vi "Main_0.2v.vi"(0 "START":bool) -> ()   [LabVIEW 2016]
uses:
  ctl/config_ctl.ctl
  ctl/force_sensor_data.ctl
  ctl/UI_cmd-ctl.ctl
  ctl/Data_buf_cmd.ctl
  ctl/file_path-cmd.ctl
  Global.vi
panel:
  out "큐의 원소 개수":i32
  out "simulation":bool
  in  "sub_tab":enum32{"graph", "ref", "err"}(tab)=enum."ref"
  in  "Grapb_tap":enum32{"data graph", "sub graph"}(tab)=enum."sub graph"
  out "Strain chart w cal":waveform(dbl)[](graph)
  out "Force chart":waveform(dbl)(graph)
  out "vacuum chart":waveform(dbl)(graph)
  out "Heater chart":i32(graph)=2147483647
  out "Strain raw chart":waveform(dbl)[](graph)=[{"t0"=timestamp(3479370102.41062 s since 1904-01-01), "dt"=0.00062, "Y"=[0.0, 0.0, 0.0, 0.0, 0.0, 0.0, 0.0, 0.0, 0.0, 0.0, 0.0, 0.0, 0.0, 0.0, 0.0, 0.0, 0.0, 0.0, 0.0, 0.0, 0.0, 0.0, 0.0, 0.0, 0.0, 0.0, 0.0, 0.0, 0.0, 0.0, 0.0, 0.0, 0.0, 0.0, 0.0, 0.0, 0.0, 0.0, 0.0, 0.0, 0.0, 0.0, 0.0, 0.0, 0.0, 0.0, 0.0, 0.0, 0.0, 0.0, 0.0, 0.0, 0.0, 0.0, 0.0, 0.0, 0.0, 0.0, 0.0, 0.0, 0.0, 0.0, 0.0, 0.0, 0.0, 0.0, 0.0, 0.0, 0.0, 0.0, 0.0, 0.0, 0.0, 0.0, 0.0, 0.0, 0.0, 0.0, 0.0, 0.0, 0.0, 0.0, 0.0, 0.0, 0.0, 0.0, 0.0, 0.0, 0.0, 0.0, 0.0, 0.0, 0.0, 0.0, 0.0, 0.0, 0.0, 0.0, 0.0, 0.0], "attributes"=variant("NI_ChannelName"=variant(string "변형률_0"), "NI_UnitDescription"=variant(string "Strain"))}, {"t0"=timestamp(3479370102.41062 s since 1904-01-01), "dt"=0.00062, "Y"=[0.0, 0.0, 0.0, 0.0, 0.0, 0.0, 0.0, 0.0, 0.0, 0.0, 0.0, 0.0, 0.0, 0.0, 0.0, 0.0, 0.0, 0.0, 0.0, 0.0, 0.0, 0.0, 0.0, 0.0, 0.0, 0.0, 0.0, 0.0, 0.0, 0.0, 0.0, 0.0, 0.0, 0.0, 0.0, 0.0, 0.0, 0.0, 0.0, 0.0, 0.0, 0.0, 0.0, 0.0, 0.0, 0.0, 0.0, 0.0, 0.0, 0.0, 0.0, 0.0, 0.0, 0.0, 0.0, 0.0, 0.0, 0.0, 0.0, 0.0, 0.0, 0.0, 0.0, 0.0, 0.0, 0.0, 0.0, 0.0, 0.0, 0.0, 0.0, 0.0, 0.0, 0.0, 0.0, 0.0, 0.0, 0.0, 0.0, 0.0, 0.0, 0.0, 0.0, 0.0, 0.0, 0.0, 0.0, 0.0, 0.0, 0.0, 0.0, 0.0, 0.0, 0.0, 0.0, 0.0, 0.0, 0.0, 0.0, 0.0], "attributes"=variant("NI_ChannelName"=variant(string "변형률_1"), "NI_UnitDescription"=variant(string "Strain"))}, {"t0"=timestamp(3479370102.41062 s since 1904-01-01), "dt"=0.00062, "Y"=[0.0, 0.0, 0.0, 0.0, 0.0, 0.0, 0.0, 0.0, 0.0, 0.0, 0.0, 0.0, 0.0, 0.0, 0.0, 0.0, 0.0, 0.0, 0.0, 0.0, 0.0, 0.0, 0.0, 0.0, 0.0, 0.0, 0.0, 0.0, 0.0, 0.0, 0.0, 0.0, 0.0, 0.0, 0.0, 0.0, 0.0, 0.0, 0.0, 0.0, 0.0, 0.0, 0.0, 0.0, 0.0, 0.0, 0.0, 0.0, 0.0, 0.0, 0.0, 0.0, 0.0, 0.0, 0.0, 0.0, 0.0, 0.0, 0.0, 0.0, 0.0, 0.0, 0.0, 0.0, 0.0, 0.0, 0.0, 0.0, 0.0, 0.0, 0.0, 0.0, 0.0, 0.0, 0.0, 0.0, 0.0, 0.0, 0.0, 0.0, 0.0, 0.0, 0.0, 0.0, 0.0, 0.0, 0.0, 0.0, 0.0, 0.0, 0.0, 0.0, 0.0, 0.0, 0.0, 0.0, 0.0, 0.0, 0.0, 0.0], "attributes"=variant("NI_ChannelName"=variant(string "변형률_2"), "NI_UnitDescription"=variant(string "Strain"))}, {"t0"=timestamp(3479370102.41062 s since 1904-01-01), "dt"=0.00062, "Y"=[0.0, 0.0, 0.0, 0.0, 0.0, 0.0, 0.0, 0.0, 0.0, 0.0, 0.0, 0.0, 0.0, 0.0, 0.0, 0.0, 0.0, 0.0, 0.0, 0.0, 0.0, 0.0, 0.0, 0.0, 0.0, 0.0, 0.0, 0.0, 0.0, 0.0, 0.0, 0.0, 0.0, 0.0, 0.0, 0.0, 0.0, 0.0, 0.0, 0.0, 0.0, 0.0, 0.0, 0.0, 0.0, 0.0, 0.0, 0.0, 0.0, 0.0, 0.0, 0.0, 0.0, 0.0, 0.0, 0.0, 0.0, 0.0, 0.0, 0.0, 0.0, 0.0, 0.0, 0.0, 0.0, 0.0, 0.0, 0.0, 0.0, 0.0, 0.0, 0.0, 0.0, 0.0, 0.0, 0.0, 0.0, 0.0, 0.0, 0.0, 0.0, 0.0, 0.0, 0.0, 0.0, 0.0, 0.0, 0.0, 0.0, 0.0, 0.0, 0.0, 0.0, 0.0, 0.0, 0.0, 0.0, 0.0, 0.0, 0.0], "attributes"=variant("NI_ChannelName"=variant(string "변형률_3"), "NI_UnitDescription"=variant(string "Strain"))}]
  out "Strain raw graph":waveform(dbl)[](graph)=[{"t0"=timestamp(3479370102.41062 s since 1904-01-01), "dt"=0.00062, "Y"=[0.04635468247337127, 0.04635468247337127, 0.04635468247337127, 0.04635468247337127, 0.04635468247337127, 0.04635468247337127, 0.04635468247337127, 0.04635468247337127, 0.04635468247337127, 0.04635468247337127, 0.04635468247337127, 0.04635468247337127, 0.04635468247337127, 0.04635468247337127, 0.04635468247337127, 0.04635468247337127, 0.04635468247337127, 0.04635468247337127, 0.04635468247337127, 0.04635468247337127, 0.04635468247337127, 0.04635468247337127, 0.04635468247337127, 0.04635468247337127, 0.04635468247337127, 0.04635468247337127, 0.04635468247337127, 0.04635468247337127, 0.04635468247337127, 0.04635468247337127, 0.04635468247337127, 0.04635468247337127, 0.04635468247337127, 0.04635468247337127, 0.04635468247337127, 0.04635468247337127, 0.04635468247337127, 0.04635468247337127, 0.04635468247337127, 0.04635468247337127, 0.04635468247337127, 0.04635468247337127, 0.04635468247337127, 0.04635468247337127, 0.04635468247337127, 0.04635468247337127, 0.04635468247337127, 0.04635468247337127, 0.04635468247337127, 0.04635468247337127, 0.04635468247337127, 0.04635468247337127, 0.04635468247337127, 0.04635468247337127, 0.04635468247337127, 0.04635468247337127, 0.04635468247337127, 0.04635468247337127, 0.04635468247337127, 0.04635468247337127, 0.04635468247337127, 0.04635468247337127, 0.04635468247337127, 0.04635468247337127, 0.04635468247337127, 0.04635468247337127, 0.04635468247337127, 0.04635468247337127, 0.04635468247337127, 0.04635468247337127, 0.04635468247337127, 0.04635468247337127, 0.04635468247337127, 0.04635468247337127, 0.04635468247337127, 0.04635468247337127, 0.04635468247337127, 0.04635468247337127, 0.04635468247337127, 0.04635468247337127, 0.04635468247337127, 0.04635468247337127, 0.04635468247337127, 0.04635468247337127, 0.04635468247337127, 0.04635468247337127, 0.04635468247337127, 0.04635468247337127, 0.04635468247337127, 0.04635468247337127, 0.04635468247337127, 0.04635468247337127, 0.04635468247337127, 0.04635468247337127, 0.04635468247337127, 0.04635468247337127, 0.04635468247337127, 0.04635468247337127, 0.04635468247337127, 0.04635468247337127], "attributes"=variant("NI_ChannelName"=variant(string "변형률_0"), "NI_UnitDescription"=variant(string "Strain"))}, {"t0"=timestamp(3479370102.41062 s since 1904-01-01), "dt"=0.00062, "Y"=[0.04702815089622699, 0.04702815089622699, 0.04702815089622699, 0.04702815089622699, 0.04702815089622699, 0.04702815089622699, 0.04702815089622699, 0.04702815089622699, 0.04702815089622699, 0.04702815089622699, 0.04702815089622699, 0.04702815089622699, 0.04702815089622699, 0.04702815089622699, 0.04702815089622699, 0.04702815089622699, 0.04702815089622699, 0.04702815089622699, 0.04702815089622699, 0.04702815089622699, 0.04702815089622699, 0.04702815089622699, 0.04702815089622699, 0.04702815089622699, 0.04702815089622699, 0.04702815089622699, 0.04702815089622699, 0.04702815089622699, 0.04702815089622699, 0.04702815089622699, 0.04702815089622699, 0.04702815089622699, 0.04702815089622699, 0.04702815089622699, 0.04702815089622699, 0.04702815089622699, 0.04702815089622699, 0.04702815089622699, 0.04702815089622699, 0.04702815089622699, 0.04702815089622699, 0.04702815089622699, 0.04702815089622699, 0.04702815089622699, 0.04702815089622699, 0.04702815089622699, 0.04702815089622699, 0.04702815089622699, 0.04702815089622699, 0.04702815089622699, 0.04702815089622699, 0.04702815089622699, 0.04702815089622699, 0.04702815089622699, 0.04702815089622699, 0.04702815089622699, 0.04702815089622699, 0.04702815089622699, 0.04702815089622699, 0.04702815089622699, 0.04702815089622699, 0.04702815089622699, 0.04702815089622699, 0.04702815089622699, 0.04702815089622699, 0.04702815089622699, 0.04702815089622699, 0.04702815089622699, 0.04702815089622699, 0.04702815089622699, 0.04702815089622699, 0.04702815089622699, 0.04702815089622699, 0.04702815089622699, 0.04702815089622699, 0.04702815089622699, 0.04702815089622699, 0.04702815089622699, 0.04702815089622699, 0.04702815089622699, 0.04702815089622699, 0.04702815089622699, 0.04702815089622699, 0.04702815089622699, 0.04702815089622699, 0.04702815089622699, 0.04702815089622699, 0.04702815089622699, 0.04702815089622699, 0.04702815089622699, 0.04702815089622699, 0.04702815089622699, 0.04702815089622699, 0.04702815089622699, 0.04702815089622699, 0.04702815089622699, 0.04702815089622699, 0.04702815089622699, 0.04702815089622699, 0.04702815089622699], "attributes"=variant("NI_ChannelName"=variant(string "변형률_1"), "NI_UnitDescription"=variant(string "Strain"))}, {"t0"=timestamp(3479370102.41062 s since 1904-01-01), "dt"=0.00062, "Y"=[0.046751224408544026, 0.046751224408544026, 0.046751224408544026, 0.046751224408544026, 0.046751224408544026, 0.046751224408544026, 0.046751224408544026, 0.046751224408544026, 0.046751224408544026, 0.046751224408544026, 0.046751224408544026, 0.046751224408544026, 0.046751224408544026, 0.046751224408544026, 0.046751224408544026, 0.046751224408544026, 0.046751224408544026, 0.046751224408544026, 0.046751224408544026, 0.046751224408544026, 0.046751224408544026, 0.046751224408544026, 0.046751224408544026, 0.046751224408544026, 0.046751224408544026, 0.046751224408544026, 0.046751224408544026, 0.046751224408544026, 0.046751224408544026, 0.046751224408544026, 0.046751224408544026, 0.046751224408544026, 0.046751224408544026, 0.046751224408544026, 0.046751224408544026, 0.046751224408544026, 0.046751224408544026, 0.046751224408544026, 0.046751224408544026, 0.046751224408544026, 0.046751224408544026, 0.046751224408544026, 0.046751224408544026, 0.046751224408544026, 0.046751224408544026, 0.046751224408544026, 0.046751224408544026, 0.046751224408544026, 0.046751224408544026, 0.046751224408544026, 0.046751224408544026, 0.046751224408544026, 0.046751224408544026, 0.046751224408544026, 0.046751224408544026, 0.046751224408544026, 0.046751224408544026, 0.046751224408544026, 0.046751224408544026, 0.046751224408544026, 0.046751224408544026, 0.046751224408544026, 0.046751224408544026, 0.046751224408544026, 0.046751224408544026, 0.046751224408544026, 0.046751224408544026, 0.046751224408544026, 0.046751224408544026, 0.046751224408544026, 0.046751224408544026, 0.046751224408544026, 0.046751224408544026, 0.046751224408544026, 0.046751224408544026, 0.046751224408544026, 0.046751224408544026, 0.046751224408544026, 0.046751224408544026, 0.046751224408544026, 0.046751224408544026, 0.046751224408544026, 0.046751224408544026, 0.046751224408544026, 0.046751224408544026, 0.046751224408544026, 0.046751224408544026, 0.046751224408544026, 0.046751224408544026, 0.046751224408544026, 0.046751224408544026, 0.046751224408544026, 0.046751224408544026, 0.046751224408544026, 0.046751224408544026, 0.046751224408544026, 0.046751224408544026, 0.046751224408544026, 0.046751224408544026, 0.046751224408544026], "attributes"=variant("NI_ChannelName"=variant(string "변형률_2"), "NI_UnitDescription"=variant(string "Strain"))}, {"t0"=timestamp(3479370102.41062 s since 1904-01-01), "dt"=0.00062, "Y"=[0.04725649492680068, 0.04725649492680068, 0.04725649492680068, 0.04725649492680068, 0.04725649492680068, 0.04725649492680068, 0.04725649492680068, 0.04725649492680068, 0.04725649492680068, 0.04725649492680068, 0.04725649492680068, 0.04725649492680068, 0.04725649492680068, 0.04725649492680068, 0.04725649492680068, 0.04725649492680068, 0.04725649492680068, 0.04725649492680068, 0.04725649492680068, 0.04725649492680068, 0.04725649492680068, 0.04725649492680068, 0.04725649492680068, 0.04725649492680068, 0.04725649492680068, 0.04725649492680068, 0.04725649492680068, 0.04725649492680068, 0.04725649492680068, 0.04725649492680068, 0.04725649492680068, 0.04725649492680068, 0.04725649492680068, 0.04725649492680068, 0.04725649492680068, 0.04725649492680068, 0.04725649492680068, 0.04725649492680068, 0.04725649492680068, 0.04725649492680068, 0.04725649492680068, 0.04725649492680068, 0.04725649492680068, 0.04725649492680068, 0.04725649492680068, 0.04725649492680068, 0.04725649492680068, 0.04725649492680068, 0.04725649492680068, 0.04725649492680068, 0.04725649492680068, 0.04725649492680068, 0.04725649492680068, 0.04725649492680068, 0.04725649492680068, 0.04725649492680068, 0.04725649492680068, 0.04725649492680068, 0.04725649492680068, 0.04725649492680068, 0.04725649492680068, 0.04725649492680068, 0.04725649492680068, 0.04725649492680068, 0.04725649492680068, 0.04725649492680068, 0.04725649492680068, 0.04725649492680068, 0.04725649492680068, 0.04725649492680068, 0.04725649492680068, 0.04725649492680068, 0.04725649492680068, 0.04725649492680068, 0.04725649492680068, 0.04725649492680068, 0.04725649492680068, 0.04725649492680068, 0.04725649492680068, 0.04725649492680068, 0.04725649492680068, 0.04725649492680068, 0.04725649492680068, 0.04725649492680068, 0.04725649492680068, 0.04725649492680068, 0.04725649492680068, 0.04725649492680068, 0.04725649492680068, 0.04725649492680068, 0.04725649492680068, 0.04725649492680068, 0.04725649492680068, 0.04725649492680068, 0.04725649492680068, 0.04725649492680068, 0.04725649492680068, 0.04725649492680068, 0.04725649492680068, 0.04725649492680068], "attributes"=variant("NI_ChannelName"=variant(string "변형률_3"), "NI_UnitDescription"=variant(string "Strain"))}]
  out "Filtered force graph":waveform(dbl)[](graph)
  out "Force graph T":waveform(dbl)(graph)={"t0"=timestamp(0 s since 1904-01-01), "dt"=0.00062, "Y"=array[3100 elements]}
  out "Balance xy T_p":cluster{"X":dbl, "Y":dbl}[](graph)=[{"X"=-5.263322791327499, "Y"=0.7308526066053755}]
  out "ROI intensity":dbl[][](graph)=[[nan, nan, nan, nan], [nan, nan, nan, nan]]
  out "error out UI":errorcluster caption="error out"
  in  "Data load":bool
  in  "Nulling":bool
  in  "pause":bool
  in  "Main_tap":T1(tab)
  in  "Balance_y":dbl(slide) scale=-50.0..50.0
  in  "Balance_x":dbl(slide) scale=-50.0..50.0
  in  "collet on/off":bool=TRUE
  out "Vacuum":dbl(knob)=27.578726717744516 scale=-10.0..80.0
  out "PCB temp":dbl[](array[slide])=[84.21052631578948, 126.31578947368422, 126.31578947368422, 126.31578947368422, 90.0, 84.21052631578948] scale=0.0..200.0
  in  "PCB config":u16(ring)=5
  in  "Zoom":bool
  out "Forece zoom Graph":dbl[](graph)
  out "simulation status":u32(slide) scale=0.0..565.1360644575578
  in  "Simulation config":cluster{"Raw data file path":path, "speed":u32}={"Raw data file path"=path "C:/FDCdata/data/*.dat", "speed"=10} {"speed" scale=0.0..100.0}
  out "Force graph T":waveform(dbl)(graph)={"t0"=timestamp(0 s since 1904-01-01), "dt"=0.00062, "Y"=array[4800 elements]}
  out "trigger":bool
  out "Pickup force":dbl=98.25510170952174 caption="Pickup force (g)" format="%.1f"
  out "Pickup time":dbl=100.0 caption="Pickup time (ms)" format="%.1f"
  in  "Status":string="\r\n15:48:53 - system ini start\r\n15:48:53 - system ini finish\r\n15:48:55 - cam ini\r\n15:49:19 - cam start\r\n15:49:20 - Program stop\r\n15:49:20 - cam stop"
  out "Balance xy rt":cluster{"X":dbl, "Y":dbl}[](graph)
  out "Bonding force":dbl=992.5036050877534 caption="Bonding force (g)" format="%.1f"
  out "Bonding time":dbl=1024.8600000000001 caption="Bonding time (ms)" format="%.1f"
  out "Heater_rt":dbl=nan caption="Heater (c)" format="%.1f"
  out "Vacuum_rt":dbl=nan caption="Vacuum (kpa)" format="%.1f"
  out "Force rt":dbl=-260.0 caption="Force(g)" format="%.1f"
  out "vacuum T":dbl=36.062310289230055 format="%.1f"
  out "Heater temp T":dbl=85.0 caption="Heater temp (dg)" format="%.1f"
  out "Detach force":dbl=35.0820285944681 caption="Detach force (g)" format="%.1f"
  out "Balance xy T":cluster{"X":dbl, "Y":dbl}[](graph)=[{"X"=-5.263322791327499, "Y"=0.7308526066053755}]
  in  "Graph tap":enum32{"All", "IR"}(tab)
  out "Mixed signal":cluster{"force":dbl, "vacuum":dbl, "temp":dbl}(graph)
  out "IR Image":T2(plugin-control)
  in  "Data_tap":enum32{"Table", "Graph"}(tab)
  out "Data Table":string[][](table)=[["989.722772 ", " 1018.660000 ", " 129.870977 ", " 275.900000 ", " 39.437574 ", " 0.007857", "-0.075730 ", " 0.031476 ", " 0.000000 ", ""], ["1035.064263 ", " 1026.720000 ", " 141.740749 ", " 279.000000 ", " 21.594200 ", " 0.064365", "-0.070932 ", " -0.026859 ", " 0.000000 ", ""], ["953.326654 ", " 1018.040000 ", " 144.008701 ", " 276.520000 ", " 19.439881 ", " 0.048826", "-0.083029 ", " 0.031694 ", " 0.000000 ", ""], ["979.122812 ", " 1027.960000 ", " 140.533487 ", " 275.900000 ", " 17.521738 ", " 0.005569", "-0.069651 ", " 0.008560 ", " 0.000000 ", ""], ["1043.949852 ", " 1042.840000 ", " 134.488977 ", " 275.900000 ", " 13.192071 ", " 0.021168", "-0.072055 ", " 0.031519 ", " 0.000000 ", ""], ["1071.984719 ", " 1048.420000 ", " 138.327061 ", " 275.280000 ", " 25.559397 ", " 0.035083", "-0.035856 ", " -0.018712 ", " 0.000000 ", ""], ["1046.754193 ", " 1028.580000 ", " 142.008722 ", " 275.900000 ", " 18.790541 ", " 0.050977", "-0.061814 ", " 0.072167 ", " 0.000000 ", ""], ["978.664436 ", " 1027.960000 ", " 136.487201 ", " 276.520000 ", " 9.468253 ", " -0.003054", "-0.055865 ", " 0.026074 ", " 0.000000 ", ""], ["976.067518 ", " 1033.540000 ", " 146.571229 ", " 276.520000 ", " 22.608603 ", " 0.020801", "-0.074720 ", " -0.001809 ", " 0.000000 ", ""], ["1056.774276 ", " 1018.660000 ", " 147.195488 ", " 273.420000 ", " 10.587437 ", " 0.032608", "-0.051327 ", " 0.007079 ", " 0.000000 ", ""], ["990.239962 ", " 1018.660000 ", " 112.936811 ", " 270.320000 ", " 42.850519 ", " 0.033952", "-0.070209 ", " 0.070206 ", " 0.000000 ", ""], ["936.169153 ", " 1018.660000 ", " 140.782457 ", " 272.800000 ", " 12.421586 ", " -0.020109", "-0.070449 ", " 0.014964 ", " 0.000000 ", ""], ["941.421956 ", " 1014.320000 ", " 149.172818 ", " 274.660000 ", " 26.213624 ", " -0.007032", "-0.073163 ", " 0.004508 ", " 0.000000 ", ""], ["1034.387749 ", " 1023.000000 ", " 138.956480 ", " 270.940000 ", " 11.759580 ", " 0.086476", "-0.084766 ", " 0.052867 ", " 0.000000 ", ""], ["996.857727 ", " 1021.760000 ", " 157.070597 ", " 274.040000 ", " 25.263497 ", " 0.047311", "-0.063551 ", " 0.014572 ", " 0.000000 ", ""], ["989.722772 ", " 1018.660000 ", " 129.870977 ", " 275.900000 ", " 39.437574 ", " 0.007857", "-0.075730 ", " 0.031476 ", " 0.000000 ", ""], ["1035.064263 ", " 1026.720000 ", " 141.740749 ", " 279.000000 ", " 21.594200 ", " 0.064365", "-0.070932 ", " -0.026859 ", " 0.000000 ", ""], ["953.326654 ", " 1018.040000 ", " 144.008701 ", " 276.520000 ", " 19.439881 ", " 0.048826", "-0.083029 ", " 0.031694 ", " 0.000000 ", ""], ["979.122812 ", " 1027.960000 ", " 140.533487 ", " 275.900000 ", " 17.521738 ", " 0.005569", "-0.069651 ", " 0.008560 ", " 0.000000 ", ""], ["1043.949852 ", " 1042.840000 ", " 134.488977 ", " 275.900000 ", " 13.192071 ", " 0.021168", "-0.072055 ", " 0.031519 ", " 0.000000 ", ""], ["1071.984719 ", " 1048.420000 ", " 138.327061 ", " 275.280000 ", " 25.559397 ", " 0.035083", "-0.035856 ", " -0.018712 ", " 0.000000 ", ""], ["1046.754193 ", " 1028.580000 ", " 142.008722 ", " 275.900000 ", " 18.790541 ", " 0.050977", "-0.061814 ", " 0.072167 ", " 0.000000 ", ""], ["978.664436 ", " 1027.960000 ", " 136.487201 ", " 276.520000 ", " 9.468253 ", " -0.003054", "-0.055865 ", " 0.026074 ", " 0.000000 ", ""], ["976.067518 ", " 1033.540000 ", " 146.571229 ", " 276.520000 ", " 22.608603 ", " 0.020801", "-0.074720 ", " -0.001809 ", " 0.000000 ", ""], ["1056.774276 ", " 1018.660000 ", " 147.195488 ", " 273.420000 ", " 10.587437 ", " 0.032608", "-0.051327 ", " 0.007079 ", " 0.000000 ", ""], ["990.239962 ", " 1018.660000 ", " 112.936811 ", " 270.320000 ", " 42.850519 ", " 0.033952", "-0.070209 ", " 0.070206 ", " 0.000000 ", ""], ["936.169153 ", " 1018.660000 ", " 140.782457 ", " 272.800000 ", " 12.421586 ", " -0.020109", "-0.070449 ", " 0.014964 ", " 0.000000 ", ""], ["941.421956 ", " 1014.320000 ", " 149.172818 ", " 274.660000 ", " 26.213624 ", " -0.007032", "-0.073163 ", " 0.004508 ", " 0.000000 ", ""], ["1034.387749 ", " 1023.000000 ", " 138.956480 ", " 270.940000 ", " 11.759580 ", " 0.086476", "-0.084766 ", " 0.052867 ", " 0.000000 ", ""], ["996.857727 ", " 1021.760000 ", " 157.070597 ", " 274.040000 ", " 25.263497 ", " 0.047311", "-0.063551 ", " 0.014572 ", " 0.000000 ", ""]]
  out "Analysis graph":dbl[](graph)
  out "Data result":cluster{"Mean":dbl, "Max":dbl, "Min":dbl}
  in  "Data menu":T3
  out "balance trend":cluster{"X":dbl, "Y":dbl}[](graph)
  in  "file path":path=path "C:/FDCdata/data/Txt-data_1429_via_simulation.txt" caption="Data file path"
  in  "config tap":enum32{"Program", "etc"}(tab)
  in  "save drive":T4(ring)
  in  "cDAQ config":T5={"sampling rate"=4000.0, "sample to read"=400.0}
  in  "Config":T6={"Lower Cut-Off"=200.0, "Vacuum Trigger level"=20.0, "state settings"={"method"=enum."histogram", "histogram size"=512, "histogram method"=enum."mode", "reserved"=1.0}, "SPA-300 Setting"={"Bonding force (g)"=1000.0, "Bonding time (ms)"=1000.0, "Pickup force (g)"=80.0, "Pickup time (ms)"=200.0, "Speed"=enum."Slow"}, "sensor file"=path ""} {"state settings"."reserved" format="%0.2f"}
  in  "Save_setting":bool
  in  "Load_setting":bool
  out "Force Sensor data":T7={"weight"={"front"=0.28, "left"=0.19, "back"=0.17, "right"=0.36}, "strain map"=[{"x"=-0.0001, "y"=-260.0}, {"x"=0.0, "y"=0.0}, {"x"=0.0001, "y"=260.0}, {"x"=0.000265, "y"=512.0}, {"x"=0.000555, "y"=1042.0}, {"x"=0.00075, "y"=1392.0}, {"x"=0.00082, "y"=1500.0}]}
  out "ROI":T8={"Global Rectangle"=[197, 225, 220, 242], "Contours"=[{"Contour Type"=0, "ROI Type"=3, "Points"=[197, 225, 220, 242]}]}
  in  "정지":bool=TRUE
  # "Real Monitoring"
  # "Balance"
  # "Force"
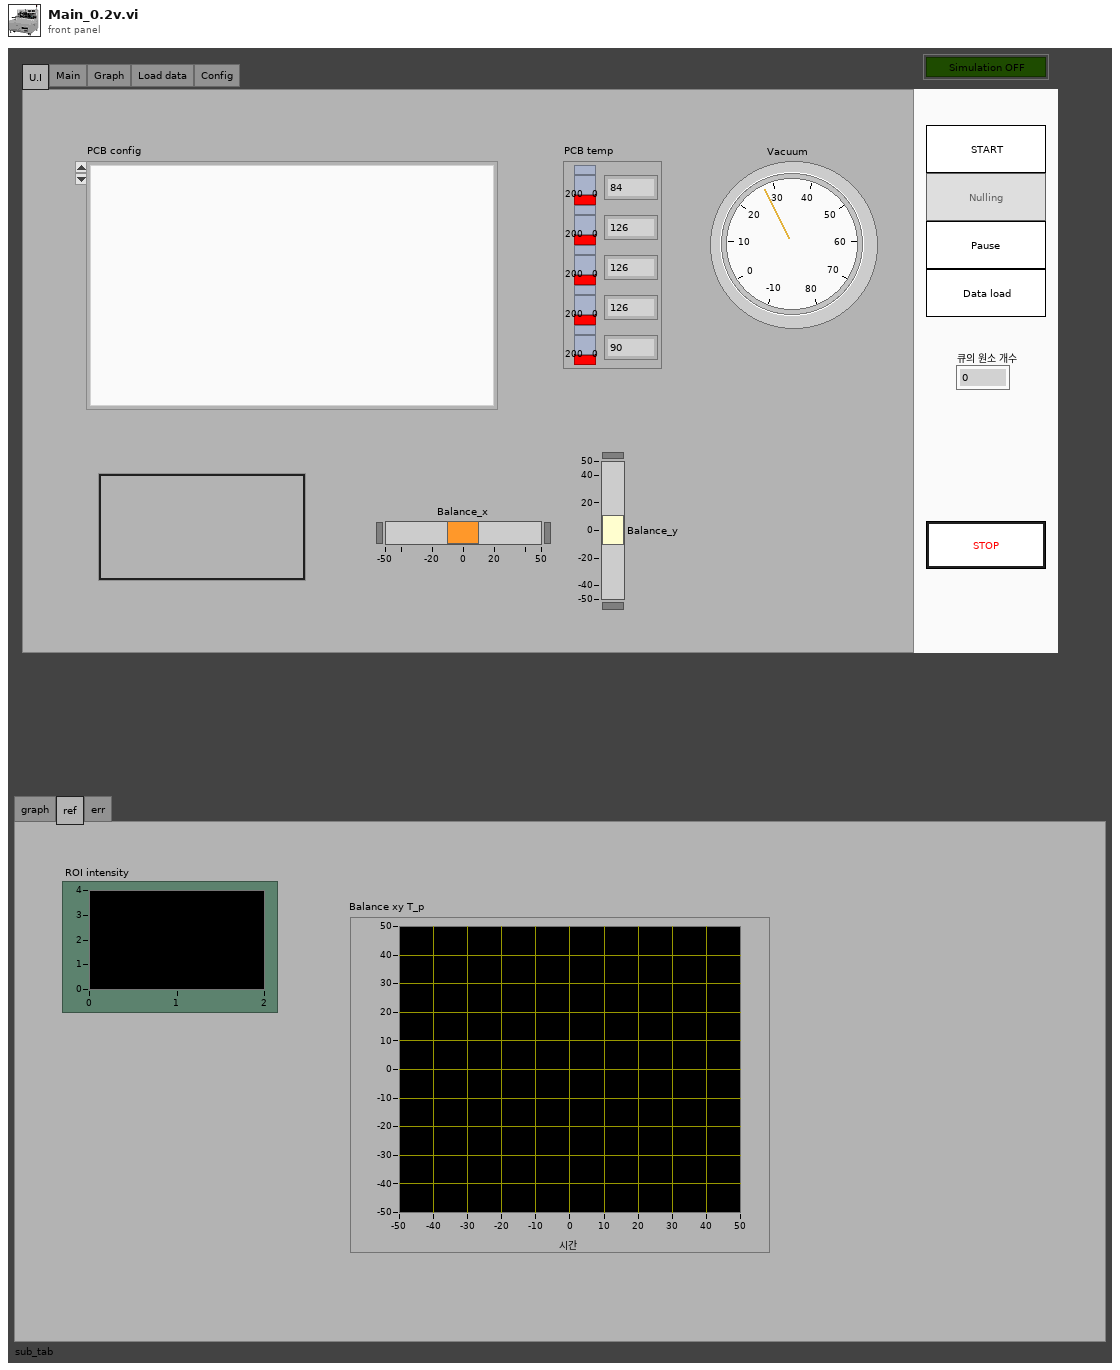
[diagram p1: front panel]
types:
  T1 = enum32{"U.I", "Main", "Graph", "Load data", "Config"}
  T2 = typedef "IMAQ Image.ctl" = refnum<image>
  T3 = cluster{"Force load":bool, "Force load 2":bool, "Force load 3":bool, "Force load 4":bool, "Force load 5":bool, "Force load 8":bool, "Force load 9":bool, "Force load 6":bool, "Force load 7":bool}
  T4 = enum16{"C:\\", "D:\\", "E:\\", "F:\\", "G:\\", "H:\\", "I:\\"}
  T5 = cluster{"sampling rate":dbl, "sample to read":dbl}
  T6 = typedef "config_ctl.ctl" = cluster{"Lower Cut-Off":dbl, "Vacuum Trigger level":dbl, "state settings":cluster{"method":enum32{"histogram", "peak", "auto select"}, "histogram size":i32, "histogram method":enum16{"mode"}, "reserved":dbl}, "SPA-300 Setting":cluster{"Bonding force (g)":dbl, "Bonding time (ms)":dbl, "Pickup force (g)":dbl, "Pickup time (ms)":dbl, "Speed":enum16{"Slow", "Fast"}}, "sensor file":path}
  T7 = typedef "force_sensor_data.ctl" = cluster{"weight":cluster{"front":dbl, "left":dbl, "back":dbl, "right":dbl}, "strain map":cluster{"x":dbl, "y":dbl}[]}
  T8 = cluster{"Global Rectangle":i32[], "Contours":cluster{"Contour Type":u32, "ROI Type":u32, "Points":i32[]}[]}
  T9 = typedef "UI_cmd-ctl.ctl" = enum16{"default", "create", "read"}
  T10 = typedef "Data_buf_cmd.ctl" = enum16{"insert", "default", "create", "clear"}
  T11 = enum8{"Enabled", "Disabled", "Disabled and Grayed Out"}
  T12 = cluster{"PCB temp":refnum<vi>, "Vacuum":refnum<vi>, "PCB config":refnum<vi>, "Balance_x":refnum<vi>, "Balance_y":refnum<vi>}
  T13 = cluster{"Heater temp T":refnum<vi>, "Heater chart":refnum<vi>, "vacuum T":refnum<vi>, "Balance xy rt":refnum<vi>, "Strain chart w cal":refnum<vi>, "Pickup force":refnum<vi>, "Pickup time":refnum<vi>, "Force chart":refnum<vi>, "Force graph T":refnum<vi>, "vacuum chart":refnum<vi>, "vacuum rt":refnum<vi>, "Strain raw graph":refnum<vi>, "Strain raw chart":refnum<vi>, "Bonding time":refnum<vi>, "Bonding force":refnum<vi>, "Balance xy T":refnum<vi>, "Filtered force graph":refnum<vi>, "ROI intensity":refnum<vi>, "Heater_rt":refnum<vi>, "Detach force":refnum<vi>, "Force rt":refnum<vi>, "Mixed signal":refnum<vi>}
  T14 = typedef "q_data.ctl" = cluster{"Strain raw wf":waveform(dbl)[], "vacuum raw wf":waveform(dbl), "IR raw 2d":i16[][]}
  T15 = typedef "log_data.ctl" = cluster{"strain filter_n_nulling wf":waveform(dbl)[], "force wf":waveform(dbl), "force":dbl, "Balance xy wfs":cluster{"X":dbl, "Y":dbl}[], "vacuum kpa wf":waveform(dbl), "pcb temp":dbl[][]}
  T16 = typedef "data.ctl" = cluster{"Bonding force":dbl, "Bonding time":dbl, "Bonding index":dbl, "Pickup force":dbl, "Pickup time":dbl, "Pickup index":dbl, "Detach force":dbl, "Detach time":dbl, "Detach index":dbl, "Heater temp rt":dbl, "Vacuum rt":dbl, "IR raw data":i16[][], "IR temp data":dbl[][], "vacuum raw wf":waveform(dbl), "vacuum kpa wf":waveform(dbl), "strain raw wf":waveform(dbl)[], "Force rt":dbl, "Vacuum T":dbl, "Heater temp T":dbl, "Balance xy arrays":cluster{dbl, dbl}[], "Balance xy":cluster{dbl, dbl}[], "Bonding wf index":dbl, "Pickup wf index":dbl, "Bonding rising index":dbl, "Bonding falling index":dbl, "Pickup rising index":dbl, "Pickup falling index":dbl}
  T17 = typedef "file_path-cmd.ctl" = enum16{"default", "write"}
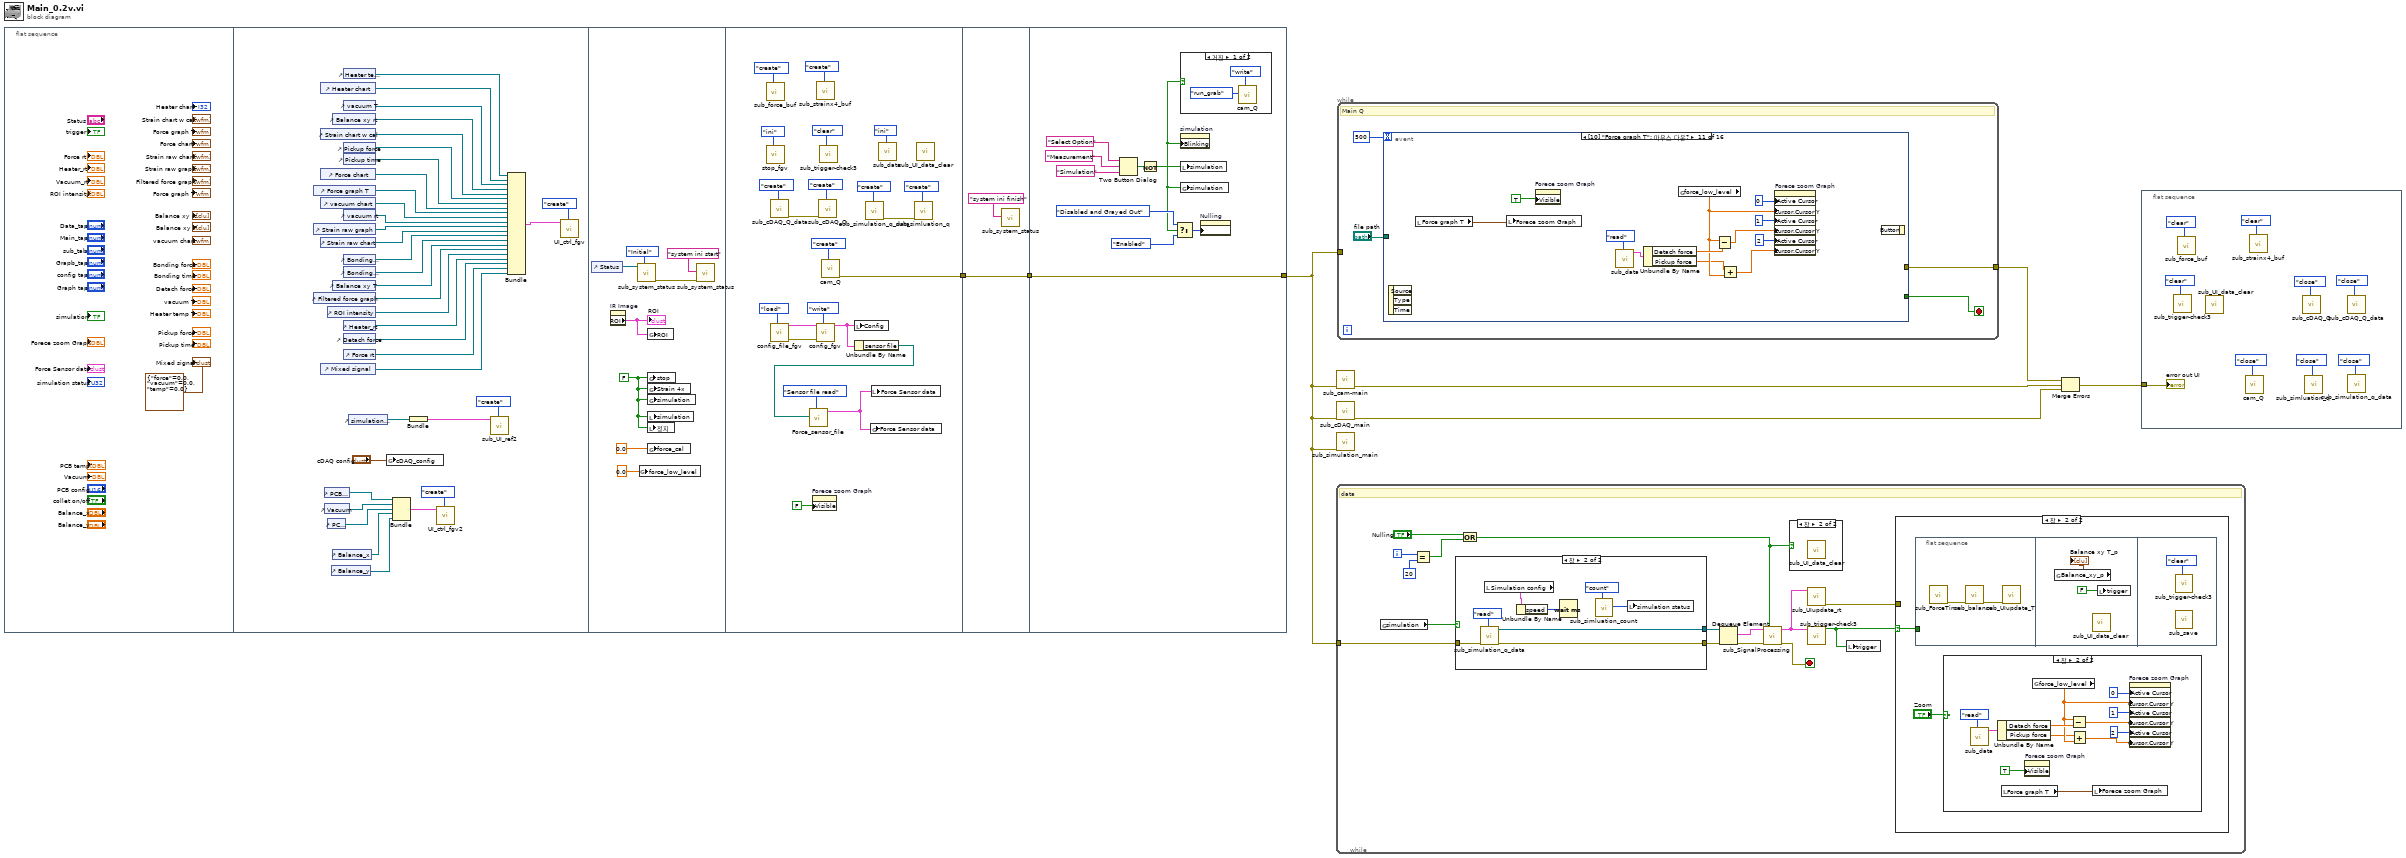
[diagram p0: block diagram]
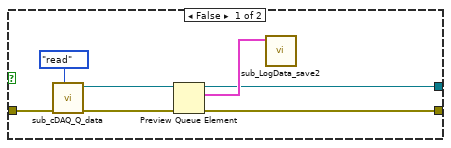
[diagram p2: hidden frame]
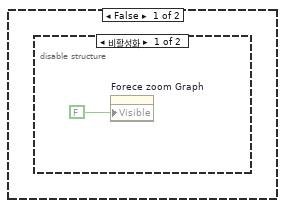
[diagram p5: hidden frame]
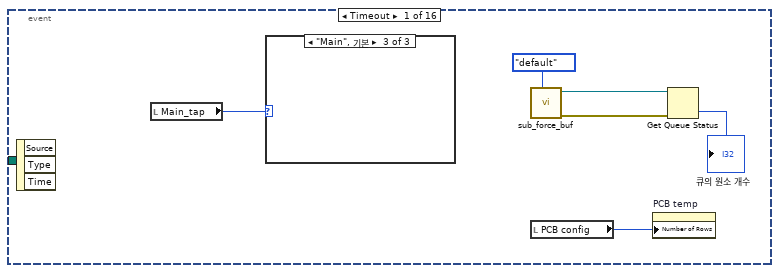
[diagram p7: hidden frame]
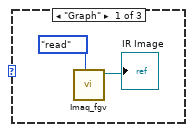
[diagram p8: hidden frame]
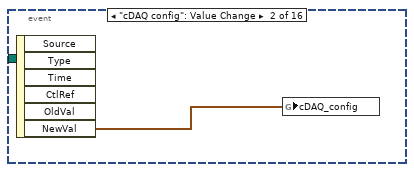
[diagram p10: hidden frame]
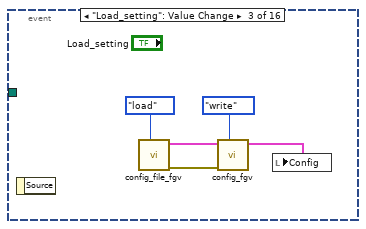
[diagram p11: hidden frame]
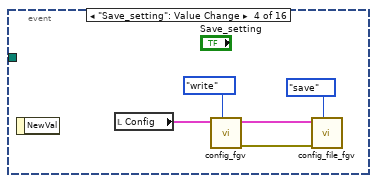
[diagram p12: hidden frame]
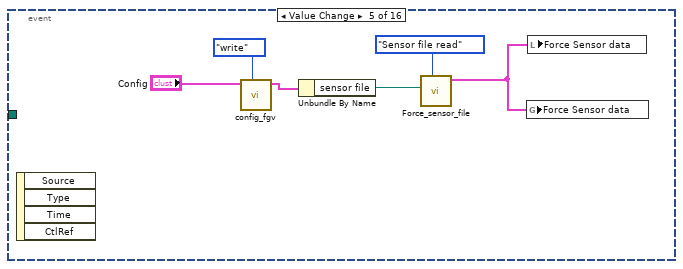
[diagram p13: hidden frame]
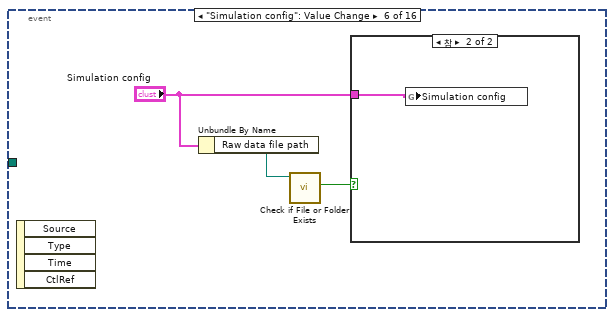
[diagram p14: hidden frame]
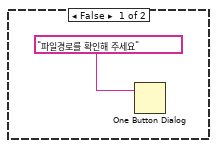
[diagram p15: hidden frame]
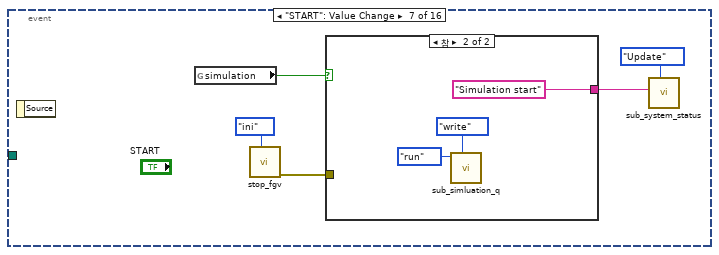
[diagram p16: hidden frame]
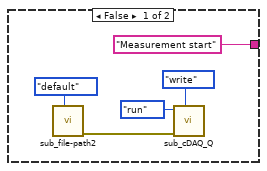
[diagram p17: hidden frame]
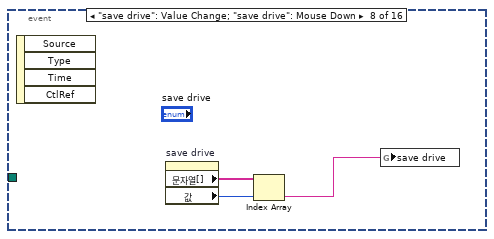
[diagram p18: hidden frame]
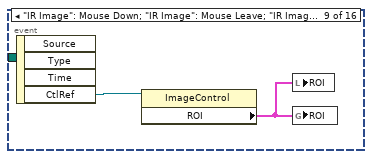
[diagram p19: hidden frame]
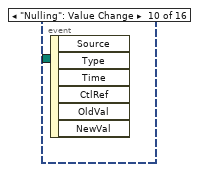
[diagram p20: hidden frame]
diagram:
  n1 = flat-sequence {
    tunnel: [w65] -> w7
    tunnel: w7 -> [w75]
    tunnel: [w75] -> w3
    tunnel: [w84] -> w4
    tunnel: w3 -> [w84]
    frame #0 {
      "Mixed signal" <- cluster{"force":dbl, "vacuum":dbl, "temp":dbl} {"force"=0.0, "vacuum"=0.0, "temp"=0.0}
    }
    frame #1 {
      n2 = control-ref of="Force graph T"() -> (w31:refnum<vi>)
      n3 = control-ref of="Strain raw graph"() -> (w41:refnum<vi>)
      n4 = control-ref of="Filtered force graph"() -> (w36:refnum<vi>)
      n5 = control-ref of="Heater chart"() -> (w24:refnum<vi>)
      n6 = control-ref of="Strain chart w cal"() -> (w27:refnum<vi>)
      n7 = control-ref of="Force chart"() -> (w30:refnum<vi>)
      n8 = control-ref of="vacuum chart"() -> (w43:refnum<vi>)
      n9 = control-ref of="Strain raw chart"() -> (w40:refnum<vi>)
      n10 = control-ref of="Mixed signal"() -> (w21:refnum<vi>)
      n11 = control-ref of="PCB temp"() -> (w13:refnum<vi>)
      n12 = control-ref of="Vacuum"() -> (w14:refnum<vi>)
      n13 = control-ref of="ROI intensity"() -> (w34:refnum<vi>)
      n14 = control-ref of="PCB config"() -> (w15:refnum<vi>)
      n15 = control-ref of="Balance_y"() -> (w10:refnum<vi>)
      n16 = control-ref of="Balance_x"() -> (w11:refnum<vi>)
      n17 = control-ref of="Balance xy rt"() -> (w26:refnum<vi>)
      n18 = control-ref of="Balance xy T"() -> (w37:refnum<vi>)
      n19 = control-ref of="Heater temp T"() -> (w23:refnum<vi>)
      n20 = control-ref of="vacuum T"() -> (w25:refnum<vi>)
      n21 = control-ref of="Pickup force"() -> (w29:refnum<vi>)
      n22 = control-ref of="Pickup time"() -> (w28:refnum<vi>)
      n23 = control-ref of="vacuum rt"() -> (w42:refnum<vi>)
      n24 = control-ref of="Bonding time"() -> (w39:refnum<vi>)
      n25 = control-ref of="Bonding force"() -> (w38:refnum<vi>)
      n26 = control-ref of="Heater_rt"() -> (w35:refnum<vi>)
      n27 = control-ref of="Detach force"() -> (w32:refnum<vi>)
      n28 = control-ref of="Force rt"() -> (w22:refnum<vi>)
      n29 = control-ref of="simulation status"() -> (w18:refnum<vi>)
      n30 = global write "Global.vi" "cDAQ_config"("cDAQ config") -> ()
      n31 = Bundle("PCB temp"=w13, "Vacuum"=w14, "PCB config"=w15, "Balance_x"=w11, "Balance_y"=w10) -> (w9:T12)  [unwired: 1 in]
      n32 = Bundle("simulation status"=w18) -> (w17:cluster{"simulation status":refnum<vi>})  [unwired: 1 in]
      n33 = call "UI_ctrl_fgv2.vi"("cmd"=enum16{"read", "create"}."create", "UI in"=w9) -> ()  [unwired: 9 in, 1 out]
      n34 = call "sub_UI_ref2.vi"("cmd"=UI_cmd-ctl."create", "UI ctl2 in"=w17) -> ()  [unwired: 9 in, 1 out]
      n35 = Bundle("Heater temp T"=w23, "Heater chart"=w24, "vacuum T"=w25, "Balance xy rt"=w26, "Strain chart w cal"=w27, "Pickup force"=w29, "Pickup time"=w28, "Force chart"=w30, "Force graph T"=w31, "vacuum chart"=w43, "vacuum rt"=w42, "Strain raw graph"=w41, "Strain raw chart"=w40, "Bonding time"=w39, "Bonding force"=w38, "Balance xy T"=w37, "Filtered force graph"=w36, "ROI intensity"=w34, "Heater_rt"=w35, "Detach force"=w32, "Force rt"=w22, "Mixed signal"=w21) -> (w20:T13)  [unwired: 1 in]
      n36 = call "UI_ctrl_fgv.vi"("cmd"=UI_cmd-ctl."create", "UI cluster in"=w20) -> ()  [unwired: 9 in, 1 out]
    }
    frame #2 {
      w45 = FALSE ("stop")
      n37 = control-ref of="Status"() -> (w50:refnum<vi>)
      n38 = property on="IR Image" class="ImageControl"() -> ("ROI"=w51:T8)  [unwired: 2 in, 2 out]
      "ROI" <- w51
      n39 = call "sub_system_status.vi"("Mode"=enum16{"Initial", "Update", "Clear"}."Initial", "System Log"=w50) -> ("에러 출력"=w48:errorcluster)  [unwired: 9 in]
      n40 = global write "Global.vi" "force_low_level"(0.0 ("force_cal")) -> ()
      n41 = global write "Global.vi" "stop"(w45) -> ()
      n42 = local write "정지"(w45) -> ()
      n43 = global write "Global.vi" "ROI"(w51) -> ()
      n44 = global write "Global.vi" "Strain 4x"(w45) -> ()
      n45 = global write "Global.vi" "simulation"(w45) -> ()
      n46 = local write "simulation"(w45) -> ()
      n47 = global write "Global.vi" "force_cal"(0.0 ("force_cal")) -> ()
      n48 = call "sub_system_status.vi"("에러 입력(에러 없음)"=w48, "String in"="system ini start") -> ()  [unwired: 9 in, 1 out]
    }
    frame #3 {
      n49 = call "sub_force_buf.vi"("cmd"=Data_buf_cmd."create") -> ()  [unwired: 9 in, 2 out]
      n50 = call "stop_fgv.vi"("cmd"=enum16{"default", "ini", "stop"}."ini") -> ()  [unwired: 9 in, 2 out]
      n51 = call "config_file_fgv.vi"("cmd"=enum16{"save", "load"}."load") -> ("error out"=w68:errorcluster, "var"=w67:T6)  [unwired: 8 in, 1 out]
      n52 = call "sub_cDAQ_Q_data.vi"("cmd"=enum16{"create", "wirte", "read", "close"}."create") -> ("error out"=w63:errorcluster)  [unwired: 9 in, 1 out]
      n53 = property on="Forece zoom Graph" class="WFGraph (엄격한)"("Visible"=FALSE ("보이기")) -> ()  [unwired: 2 in, 2 out]
      n54 = call "config_fgv.vi"("cmd"=enum16{"write", "read", "ini"}."write", "error in"=w68, "Config in"=w67) -> ("Config out"=w57:T6)  [unwired: 7 in, 1 out]
      n55 = call "sub_strainx4_buf.vi"("cmd"=Data_buf_cmd."create") -> ()  [unwired: 9 in, 2 out]
      n56 = call "sub_cDAQ_Q.vi"("cmd"=enum16{"create", "write", "read", "close"}."create", "error in"=w63) -> ()  [unwired: 8 in, 2 out]
      n57 = call "sub_trigger-check3.vi"("cmd"=enum16{"check", "clear"}."clear") -> ()  [unwired: 10 in, 1 out]
      n58 = call "cam_Q.vi"("cmd"=enum16{"create", "write", "read", "close"}."create") -> ("error out"=w65:errorcluster)  [unwired: 9 in, 1 out]
      n59 = local write "Config"(w57) -> ()
      n60 = Unbundle By Name(w57) -> ("sensor file"=w54:path)
      n61 = call "Force_sensor_file.vi"("cmd"=enum16{"Sensor file create", "Sensor file read"}."Sensor file read", "file path"=w54) -> ("Force Sensor data out"=w56:T7)  [unwired: 8 in, 1 out]
      n62 = call "sub_simulation_q_data.vi"("cmd"=enum16{"create", "wirte", "read", "close"}."create") -> ("error out"=w58:errorcluster)  [unwired: 9 in, 1 out]
      n63 = global write "Global.vi" "Force Sensor data"(w56) -> ()
      n64 = local write "Force Sensor data"(w56) -> ()
      n65 = call "sub_data.vi"("cmd"=enum16{"ini", "write", "read"}."ini") -> ()  [unwired: 9 in, 2 out]
      n66 = call "sub_simluation_q.vi"("cmd"=enum16{"create", "write", "read", "close"}."create", "error in"=w58) -> ()  [unwired: 8 in, 2 out]
      n67 = call "sub_UI_data_clear.vi"() -> ()  [unwired: 12 in]
    }
    frame #4 {
      n68 = call "sub_system_status.vi"("String in"="system ini finish") -> ()  [unwired: 10 in, 1 out]
    }
    frame #5 {
      n69 = Two Button Dialog(message="Select Option" ("메시지"), 1:"Simulation" ("참 버튼 이름(\"확인\")"), 2:"Measurement" ("거짓 버튼 이름(\"취소\")")) -> (T button?=w80:bool)
      n70 = Not(x=w80) -> (.not. x?=w76:bool)
      n71 = Select(t=T11."Disabled and Grayed Out" ("비활성화"), s=w76, f=T11."Enabled" ("비활성화")) -> (s? t:f=w79:T11)
      n72 = property on="simulation" class="Bool (엄격한)"("Blinking"=w76) -> ()  [unwired: 2 in, 2 out]
      n73 = case shown="거짓" w76 {
        frame False {
          n74 = call "cam_Q.vi"("cmd"=enum16{"create", "write", "read", "close"}."write", "data"=enum16{"run_grab", "stop"}."run_grab") -> ()  [unwired: 8 in, 2 out]
        }
        frame True {
        }
      }
      n75 = local write "simulation"(w76) -> ()
      n76 = global write "Global.vi" "simulation"(w76) -> ()
      n77 = property on="Nulling" class="Bool"("DisabledEnum"=w79) -> ()  [unwired: 2 in, 2 out]
    }
  }
  n78 = call "sub_cam-main.vi"("error in"=w4) -> ("error out"=w2:errorcluster)  [unwired: 10 in]
  n79 = call "sub_cDAQ_main.vi"("error in"=w4) -> ("error out"=w1:errorcluster)  [unwired: 10 in]
  n80 = call "sub_simulation_main.vi"("error in"=w4) -> ()  [unwired: 10 in, 1 out]
  n81 = while {
    tunnel: w4 -> [w100]
    i -> [w99]
    stop <- w101 stop-if-true
    # "data"
    n82 = global read "Global.vi" "simulation"() -> (w88:bool)
    n83 = Equal?(x=w99, y=20) -> (x = y?=w89:bool)
    n84 = case shown="참" w88 {
      tunnel: w100 -> [w108 w115]
      tunnel: [w104 w114] -> w95
      tunnel: [w102 w113] -> w94
      frame False {
        n85 = call "sub_cDAQ_Q_data.vi"("cmd"=enum16{"create", "wirte", "read", "close"}."read", "error in"=w108) -> ("error out"=w103:errorcluster, "queue out"=w106:refnum<queue>)  [unwired: 8 in]
        n86 = Preview Queue Element(queue=w106, error in (no error)=w103) -> (queue out=w104:refnum<queue>, element=w105:T14, error out=w102:errorcluster)  [unwired: 1 in, 1 out]
        n87 = call "sub_LogData_save2.vi"("Q_data"=w105) -> ()  [unwired: 10 in, 1 out]
      }
      frame True {
        n88 = call "sub_simulation_q_data.vi"("cmd"=enum16{"create", "wirte", "read", "close"}."read", "error in"=w115) -> ("error out"=w113:errorcluster, "queue out"=w114:refnum<queue>)  [unwired: 8 in]
        n89 = local read "Simulation config"() -> (w110:cluster{"Raw data file path":path, "speed":u32})
        n90 = Unbundle By Name(w110) -> ("speed"=w109:u32)
        n91 = Wait (ms)(milliseconds to wait=w109) -> ()  [unwired: 1 out]
        n92 = call "sub_simluation_count.vi"("cmd"=enum16{"ini", "count"}."count") -> ("current"=w112:u32)  [unwired: 9 in, 1 out]
        n93 = local write "simulation status"(w112) -> ()
      }
    }
    n94 = Or(x="Nulling", y=w89) -> (x .or. y?=w91:bool)
    n95 = Dequeue Element(queue=w95, error in (no error)=w94) -> (element=w92:T14, error out=w90:errorcluster)  [unwired: 1 in, 2 out]
    n96 = call "sub_SignalProcessing.vi"("nulling"=w91, "error in"=w90, "Q_data"=w92) -> ("error out"=w101:errorcluster, "log data"=w97:T15)  [unwired: 7 in]
    n97 = case shown="참" w91 {
      frame False {
      }
      frame True {
        n98 = call "sub_UI_data_clear.vi"() -> ()  [unwired: 12 in]
      }
    }
    n99 = call "sub_UIupdate_rt.vi"("log data"=w97) -> ("error out"=w87:errorcluster)  [unwired: 10 in]
    n100 = call "sub_trigger-check3.vi"("log data"=w97) -> ("trigger"=w98:bool)  [unwired: 10 in]
    n101 = local write "trigger"(w98) -> ()
    n102 = case shown="참" w98 {
      selector: w98 -> [_ w118]
      tunnel: w87 -> [_ _]
      frame False {
      }
      frame True {
        n103 = flat-sequence {
          tunnel: w118 -> [_]
          frame #0 {
            n104 = call "sub_ForceTime.vi"() -> ("error out"=w133:errorcluster)  [unwired: 10 in, 1 out]
            n105 = call "sub_balance.vi"("error in"=w133) -> ("error out"=w132:errorcluster)  [unwired: 9 in, 1 out]
            n106 = call "sub_UIupdate_T.vi"("error in"=w132) -> ()  [unwired: 10 in, 1 out]
          }
          frame #1 {
            n107 = global read "Global.vi" "Balance_xy_p"() -> (→"Balance xy T_p":cluster{dbl, dbl}[])
            n108 = call "sub_UI_data_clear.vi"() -> ()  [unwired: 12 in]
            n109 = local write "trigger"(FALSE ("trigger")) -> ()
          }
          frame #2 {
            n110 = call "sub_trigger-check3.vi"("cmd"=enum16{"check", "clear"}."clear") -> ()  [unwired: 10 in, 1 out]
            n111 = call "sub_save.vi"() -> ()  [unwired: 12 in]
          }
        }
        n112 = case shown="참" "Zoom" {
          frame False {
            n113 = disable-structure shown="비활성화" {
              frame Disabled {
                n114 = property on="Forece zoom Graph" class="WFGraph (엄격한)"("Visible"=FALSE ("보이기")) -> ()  [unwired: 2 in, 2 out]
              }
              frame Enabled {
              }
            }
          }
          frame True {
            n115 = call "sub_data.vi"("cmd"=enum16{"ini", "write", "read"}."read") -> ("data out"=w129:T16)  [unwired: 9 in, 1 out]
            n116 = Unbundle By Name(w129) -> ("Detach force"=w127:dbl, "Pickup force"=w123:dbl)
            n117 = local read "Force graph T"() -> (w121:waveform(dbl))
            n118 = property on="Forece zoom Graph" class="WFGraph (엄격한)"("Visible"=TRUE ("보이기")) -> ()  [unwired: 2 in, 2 out]
            n119 = global read "Global.vi" "force_low_level"() -> (w124:dbl)
            n120 = Subtract(x=w124, y=w127) -> (x-y=w126:dbl)
            n121 = Add(x=w123, y=w124) -> (x+y=w122:dbl)
            n122 = local write "Forece zoom Graph"(w121) -> ()
            n123 = property on="Forece zoom Graph" class="WFGraph (엄격한)"("Active Cursor"=u32 0 ("활성 커서"), "Cursor.Cursor Y"=w124, "Active Cursor"=u32 1 ("활성 플롯"), "Cursor.Cursor Y"=w126, "Active Cursor"=u32 2 ("활성 커서"), "Cursor.Cursor Y"=w122) -> ()  [unwired: 2 in, 2 out]
          }
        }
      }
    }
  }
  n124 = while {
    tunnel: w4 -> [_]
    tunnel: [w139] -> w6
    stop <- w140 stop-if-true
    # "Main Q"
    n125 = event shown="[10] \"Force graph T\": 마우스 다운?" {
      selector: _ -> [_ _ _ _ _ _ _ _ _ _ _ _ _ _ _ _]
      dyn-events: _ -> [_ _ _ _ _ _ _ _ _ _ _ _ _ _ _ _]
      timeout: 500 -> [_ _ _ _ _ _ _ _ _ _ _ _ _ _ _ _]
      tunnel: [_ _ _ _ _ _ _ _ _ _ _ _ _ _ w246 _] -> w140
      tunnel: [_ _ _ _ _ _ _ _ _ _ _ _ _ _ _ w249] -> w139
      tunnel: "file path" -> [_ _ _ _ _ _ _ _ _ _ _ _ w202 w220 _ _]
      event Timeout {
        n126 = event-data() -> ()  [unwired: 1 in, 3 out]
        n127 = local read "Main_tap"() -> (w146:T1)
        n128 = case shown="\"Main\", 기본" w146 {
          frame "Graph" {
            n129 = call "Imaq_fgv.vi"("cmd"=enum16{"create", "close", "read"}."read") -> ("New Image"=→"IR Image":T2)  [unwired: 9 in, 1 out]
          }
          frame "Load data" {
          }
          frame "Main", Default {
          }
        }
        n130 = call "sub_force_buf.vi"("cmd"=Data_buf_cmd."default") -> ("error out"=w142:errorcluster, "queue out"=w143:refnum<queue>)  [unwired: 9 in]
        n131 = local read "PCB config"() -> (w145:u16)
        n132 = property on="PCB temp" class="Arr (엄격한)"("Number of Rows"=w145) -> ()  [unwired: 2 in, 2 out]
        n133 = Get Queue Status(queue=w143, error in (no error)=w142) -> (# elements in queue=→"큐의 원소 개수":i32)  [unwired: 1 in, 7 out]
      }
      event "cDAQ config": Value Change {
        n134 = event-data() -> ("NewVal"=w149:T5)  [unwired: 1 in, 5 out]
        n135 = global write "Global.vi" "cDAQ_config"(w149) -> ()
      }
      event "Load_setting": Value Change {
        n136 = event-data() -> ()  [unwired: 1 in, 1 out]
        n137 = call "config_file_fgv.vi"("cmd"=enum16{"save", "load"}."load") -> ("error out"=w153:errorcluster, "var"=w152:T6)  [unwired: 8 in, 1 out]
        n138 = call "config_fgv.vi"("cmd"=enum16{"write", "read", "ini"}."write", "error in"=w153, "Config in"=w152) -> ("Config out"=w150:T6)  [unwired: 7 in, 1 out]
        n139 = local write "Config"(w150) -> ()
      }
      event "Save_setting": Value Change {
        n140 = event-data() -> ()  [unwired: 1 in, 1 out]
        n141 = local read "Config"() -> (w156:T6)
        n142 = call "config_fgv.vi"("cmd"=enum16{"write", "read", "ini"}."write", "Config in"=w156) -> ("error out"=w157:errorcluster, "Config out"=w155:T6)  [unwired: 8 in]
        n143 = call "config_file_fgv.vi"("cmd"=enum16{"save", "load"}."save", "error in"=w157, "Config"=w155) -> ()  [unwired: 6 in, 3 out]
      }
      event Value Change {
        n144 = event-data() -> ()  [unwired: 1 in, 4 out]
        n145 = call "config_fgv.vi"("cmd"=enum16{"write", "read", "ini"}."write", "Config in"="Config") -> ("Config out"=w163:T6)  [unwired: 8 in, 1 out]
        n146 = Unbundle By Name(w163) -> ("sensor file"=w160:path)
        n147 = call "Force_sensor_file.vi"("cmd"=enum16{"Sensor file create", "Sensor file read"}."Sensor file read", "file path"=w160) -> ("Force Sensor data out"=w161:T7)  [unwired: 8 in, 1 out]
        n148 = global write "Global.vi" "Force Sensor data"(w161) -> ()
        n149 = local write "Force Sensor data"(w161) -> ()
      }
      event "Simulation config": Value Change {
        n150 = event-data() -> ()  [unwired: 1 in, 4 out]
        n151 = Unbundle By Name("Simulation config") -> ("Raw data file path"=w168:path)
        n152 = call <vilib>:"Check if File or Folder Exists.vi"("path"=w168) -> ("file or folder exists?"=w167:bool)  [unwired: 8 in, 2 out]
        n153 = case shown="참" w167 {
          tunnel: "Simulation config" -> [_ w170]
          frame False {
            n154 = One Button Dialog(message="파일경로를 확인해 주세요" ("메시지")) -> ()  [unwired: 1 in, 1 out]
          }
          frame True {
            n155 = global write "Global.vi" "Simulation config"(w170) -> ()
          }
        }
      }
      event "START": Value Change {
        n156 = event-data() -> ()  [unwired: 1 in, 1 out]
        n157 = global read "Global.vi" "simulation"() -> (w172:bool)
        n158 = call "stop_fgv.vi"("cmd"=enum16{"default", "ini", "stop"}."ini") -> ("error out"=w173:errorcluster)  [unwired: 9 in, 1 out]
        n159 = case shown="참" w172 {
          tunnel: w173 -> [_ _]
          tunnel: ["Measurement start" ("String in") "Simulation start" ("String in")] -> w171
          frame False {
            n160 = call "sub_file-path2.vi"("cmd"=file_path-cmd."default") -> ("error out"=w176:errorcluster)  [unwired: 8 in, 2 out]
            n161 = call "sub_cDAQ_Q.vi"("cmd"=enum16{"create", "write", "read", "close"}."write", "error in"=w176, "data"=enum16{"run", "stop"}."run") -> ()  [unwired: 7 in, 2 out]
          }
          frame True {
            n162 = call "sub_simluation_q.vi"("cmd"=enum16{"create", "write", "read", "close"}."write", "data"=enum16{"run", "stop"}."run") -> ()  [unwired: 8 in, 2 out]
          }
        }
        n163 = call "sub_system_status.vi"("Mode"=enum16{"Initial", "Update", "Clear"}."Update", "String in"=w171) -> ()  [unwired: 9 in, 1 out]
      }
      event "save drive": Value Change; "save drive": Mouse Down {
        n164 = event-data() -> ()  [unwired: 1 in, 4 out]
        n165 = property on="save drive" class="Enum (엄격한)"() -> ("문자열[]"=w186:string[], "값"=w185:T4)  [unwired: 2 in, 2 out]
        n166 = Index Array(array=w186, index=w185) -> (element=w184:string)
        n167 = global write "Global.vi" "save drive"(w184) -> ()
      }
      event "IR Image": Mouse Down; "IR Image": Mouse Leave; "IR Image": Mouse Move {
        n168 = event-data() -> ("CtlRef"=w188:refnum<vi>)  [unwired: 1 in, 3 out]
        n169 = property class="ImageControl"(reference=w188) -> ("ROI"=w187:T8)  [unwired: 1 in, 2 out]
        n170 = local write "ROI"(w187) -> ()
        n171 = global write "Global.vi" "ROI"(w187) -> ()
      }
      event "Nulling": Value Change {
        n172 = event-data() -> ()  [unwired: 1 in, 6 out]
      }
      event "Force graph T": Mouse Down? {
        n173 = event-data() -> ()  [unwired: 1 in, 3 out]
        n174 = local read "Force graph T"() -> (w199:waveform(dbl))
        n175 = local write "Forece zoom Graph"(w199) -> ()
        n176 = property on="Forece zoom Graph" class="WFGraph (엄격한)"("Visible"=TRUE ("보이기")) -> ()  [unwired: 2 in, 2 out]
        n177 = call "sub_data.vi"("cmd"=enum16{"ini", "write", "read"}."read") -> ("data out"=w196:T16)  [unwired: 9 in, 1 out]
        n178 = Unbundle By Name(w196) -> ("Detach force"=w194:dbl, "Pickup force"=w190:dbl)
        n179 = global read "Global.vi" "force_low_level"() -> (w191:dbl)
        n180 = Subtract(x=w191, y=w194) -> (x-y=w193:dbl)
        n181 = Add(x=w190, y=w191) -> (x+y=w189:dbl)
        n182 = property on="Forece zoom Graph" class="WFGraph (엄격한)"("Active Cursor"=u32 0 ("활성 커서"), "Cursor.Cursor Y"=w191, "Active Cursor"=u32 1 ("활성 플롯"), "Cursor.Cursor Y"=w193, "Active Cursor"=u32 2 ("활성 커서"), "Cursor.Cursor Y"=w189) -> ()  [unwired: 2 in, 2 out]
        n183 = event-data() -> ()  [unwired: 2 in, 1 out]
      }
      event "Forece zoom Graph": Mouse Down? {
        n184 = event-data() -> ()  [unwired: 1 in, 3 out]
        n185 = property on="Forece zoom Graph" class="WFGraph (엄격한)"("Visible"=FALSE ("보이기")) -> ()  [unwired: 2 in, 2 out]
        n186 = event-data() -> ()  [unwired: 2 in, 1 out]
      }
      event "Data load": Value Change {
        n187 = event-data() -> ()  [unwired: 1 in, 3 out]
        n188 = call <vilib>:"Check if File or Folder Exists.vi"("path"=w202) -> ()  [unwired: 8 in, 3 out]
        n189 = local write "Data_tap"(enum32{"Table", "Graph"}."Table" ("Data_tap")) -> ()
      }
      event "Data menu": Value Change {
        n190 = event-data() -> ()  [unwired: 1 in, 1 out]
        n191 = Open/Create/Replace File(file path (use dialog)=w220) -> (refnum out=w213:refnum<file>, error out=w214:errorcluster)  [unwired: 5 in, 1 out]
        n192 = Read from Text File(file (use dialog)=w213, error in=w214) -> (refnum out=w211:refnum<file>, text=w210:string, error out=w212:errorcluster)  [unwired: 2 in, 1 out]
        n193 = Close File(refnum=w211, error in=w212) -> ()  [unwired: 2 out]
        n194 = Spreadsheet String To Array(format string="%f" ("format (%s)"), spreadsheet string=w210, array type (2D Dbl)=string[][] []) -> (array=w207:string[][])  [unwired: 1 in]
        n195 = Cluster To Array(cluster="Data menu") -> (array=w217:bool[])
        n196 = Index Array(array=w207) -> (element=w206:string[])  [unwired: 2 in]
        n197 = Delete From Array(array=w207, index (row)=0 ("인덱스 (행)")) -> (array with subset deleted=w215:string[][])  [unwired: 2 in, 1 out]
        n198 = Search 1D Array(1D array=w217, element=TRUE ("원소")) -> (index of element=w205:i32)  [unwired: 1 in]
        n199 = property on="Data Table" class="Tbl (엄격한)"("Column Headers[]"=w206) -> ()  [unwired: 2 in, 2 out]
        n200 = Index Array(array=w215, index (col)=w205) -> (element=w204:string[])  [unwired: 1 in]
        n201 = case shown="5" w205 {
          tunnel: w204 -> [w222 w236]
          frame 5 {
            n202 = for {
              tunnel: w222 -> [w229] mode=indexing
              tunnel: [w223] -> w221 mode=indexing
              n203 = Match Pattern(string=w229, regular expression="," ("정규식")) -> (before substring=w226:string, after substring=w227:string)  [unwired: 1 in, 2 out]
              n204 = Fract/Exp String To Number(string=w226) -> (number=w225:dbl)  [unwired: 3 in, 1 out]
              n205 = Fract/Exp String To Number(string=w227) -> (number=w224:dbl)  [unwired: 3 in, 1 out]
              n206 = Bundle(w225, w224) -> (w223:cluster{dbl, dbl})  [unwired: 1 in]
            }
            "balance trend" <- w221
          }
          frame 1, Default {
            n207 = Fract/Exp String To Number(string=w236) -> (number=w230:dbl[])  [unwired: 3 in, 1 out]
            "Analysis graph" <- w230
            n208 = Add Array Elements(numeric array=w230) -> (sum=w232:dbl)
            n209 = Array Size(array=w230) -> (size(s)=w233:i32)
            n210 = Array Max & Min(array=w230) -> (max value=w234:dbl, min value=w237:dbl)  [unwired: 2 out]
            n211 = Divide(x=w232, y=w233) -> (x/y=w231:dbl)
            n212 = Bundle(w231, w234, w237) -> (→"Data result":cluster{dbl, dbl, dbl})  [unwired: 1 in]
          }
        }
      }
      event "정지": Value Change {
        w246 = TRUE ("stop")
        n213 = event-data() -> ()  [unwired: 1 in, 1 out]
        n214 = call "stop_fgv.vi"("cmd"=enum16{"default", "ini", "stop"}."stop") -> ("error out"=w240:errorcluster)  [unwired: 9 in, 1 out]
        n215 = call "sub_simluation_q.vi"("cmd"=enum16{"create", "write", "read", "close"}."write", "data"=enum16{"run", "stop"}."stop") -> ()  [unwired: 8 in, 2 out]
        n216 = call "sub_cDAQ_Q.vi"("cmd"=enum16{"create", "write", "read", "close"}."write", "data"=enum16{"run", "stop"}."stop") -> ()  [unwired: 8 in, 2 out]
        n217 = call "cam_Q.vi"("cmd"=enum16{"create", "write", "read", "close"}."write", "error in"=w240, "data"=enum16{"run_grab", "stop"}."stop") -> ()  [unwired: 7 in, 2 out]
        n218 = global write "Global.vi" "stop"(w246) -> ()
        n219 = call "sub_system_status.vi"("String in"="Program stop") -> ()  [unwired: 10 in, 1 out]
      }
      event "pause": Value Change {
        n220 = event-data() -> ()  [unwired: 1 in, 6 out]
        n221 = property on="Nulling" class="Bool"("DisabledEnum"=T11."Enabled" ("비활성화")) -> ()  [unwired: 2 in, 2 out]
        n222 = call "stop_fgv.vi"("cmd"=enum16{"default", "ini", "stop"}."stop") -> ("error out"=w249:errorcluster)  [unwired: 9 in, 1 out]
      }
    }
  }
  n223 = Merge Errors(w6, w2, w1) -> (w5:errorcluster)
  n224 = flat-sequence {
    tunnel: w5 -> [w258]
    frame #0 {
      n225 = call "sub_trigger-check3.vi"("cmd"=enum16{"check", "clear"}."clear") -> ()  [unwired: 10 in, 1 out]
      n226 = call "sub_force_buf.vi"("cmd"=Data_buf_cmd."clear") -> ()  [unwired: 9 in, 2 out]
      n227 = call "sub_UI_data_clear.vi"() -> ()  [unwired: 12 in]
      n228 = call "cam_Q.vi"("cmd"=enum16{"create", "write", "read", "close"}."close") -> ()  [unwired: 9 in, 2 out]
      n229 = call "sub_strainx4_buf.vi"("cmd"=Data_buf_cmd."clear") -> ()  [unwired: 9 in, 2 out]
      n230 = call "sub_cDAQ_Q.vi"("cmd"=enum16{"create", "write", "read", "close"}."close") -> ()  [unwired: 9 in, 2 out]
      n231 = call "sub_simluation_q.vi"("cmd"=enum16{"create", "write", "read", "close"}."close") -> ()  [unwired: 9 in, 2 out]
      n232 = call "sub_cDAQ_Q_data.vi"("cmd"=enum16{"create", "wirte", "read", "close"}."close") -> ()  [unwired: 9 in, 2 out]
      n233 = call "sub_simulation_q_data.vi"("cmd"=enum16{"create", "wirte", "read", "close"}."close") -> ()  [unwired: 9 in, 2 out]
      "error out UI" <- w258
    }
  }
